vi "WS1050 36 DUT CP CV Sweep SubVI.vi"(0 "TMN DC\\CAP Data Log File Path":path=path "C:/WS1050 36 DUT Data", 1 "Test Program":string="WS1050 36 DUT CP CV Sweep SubVI", 3 "Lot#":string="WS1050", 4 "Wafer#":string="T7-EB", 5 "Board#":string="BRD5", 6 "Temp":string, 7 "error in (no error)":errorcluster, 8 "File Name":string="CYC_WS1050_T7_EB_65C_40V_25DC_EMPTY_BRD5_141017_1", 9 "Comment":string="CYC65C40V", 10 "Ke2400":refnum<visa-resource-name>="GPIB0::3::INSTR", 11 "PS1 Source":refnum<visa-resource-name>="GPIB0::5::INSTR", 12 "Serial Number":string[][](table)=[["DUT", "SN"], ["DUT1", "1"], ["DUT2", "2"], ["DUT3", "3"], ["DUT4", "4"], ["DUT5", "5"], ["DUT6", "6"], ["DUT7", "7"], ["DUT8", "8"], ["DUT9", "9"], ["DUT10", "10"], ["DUT11", "11"], ["DUT12", "12"], ["DUT13", "13"], ["DUT14", "14"], ["DUT15", "15"], ["DUT16", "16"], ["DUT17", "17"], ["DUT18", "18"], ["DUT19", "19"], ["DUT20", "20"], ["DUT21", "21"], ["DUT22", "22"], ["DUT23", "23"], ["DUT24", "24"], ["DUT25", "25"], ["DUT26", "26"], ["DUT27", "27"], ["DUT28", "28"], ["DUT29", "29"], ["DUT30", "30"], ["DUT31", "31"], ["DUT32", "32"], ["DUT33", "33"], ["DUT34", "34"], ["DUT35", "35"], ["DUT36", "36"]], 14 "CP Set to Run":dbl[][](array[numeric]), 16 "HD/Cycles Completed":string="Test Data", 18 "Ke2000":refnum<visa-resource-name>="GPIB0::9::INSTR") -> (13 "40V_1":string[][](table), 15 "40V_2":string[][](table), 17 "40V_3":string[][](table), 20 "Plot_1":dbl[][](graph) caption="(Y) Multi Plot 2", 21 "Plot_2":dbl[][](graph) caption="(Y) Multi Plot 2", 22 "Ke2400 Out":refnum<visa-resource-name>="GPIB0::3::INSTR", 23 "Plot_3":dbl[][](graph) caption="(Y) Multi Plot 2", 24 "CP Voltage":string, 25 "PS1 Out":refnum<visa-resource-name>, 26 "Ke2000 Out":refnum<visa-resource-name>="GPIB0::9::INSTR", 27 "error out":errorcluster)   [LabVIEW 2012]
uses:
  WS_VCAP Driver 029/Source/WSVCAP Shell/Type Defs/WSVCAP SHL I2C DUT Mask Mode Enum.ctl
panel:
  in  "Reg1_Bit Cntrl":string[](array[string])=["01", "02", "04", "08", "10", "20", "40", "80", "03", "06", "0C", "D8", "33", "66", "CC", "07", "0E", "1C", "38", "70", "E0", "0F", "1E", "3C", "78", "F0", "1F", "3E", "7C", "F8", "3F", "7E", "FC", "7F", "FE", "FD", "FB", "F7", "EF", "DF", "BF", "7F", "FC", "F9", "F3", "E7", "CF", "9F", "3F", "F8", "F1", "E3", "C7", "8F", "1F", "F0", "E1", "C3", "87", "0F", "E0", "C1", "83", "07", "C0", "81", "03", "AA", "55", "00"]
  out "date string":string="5/19/2014"
  in  "VPI_Cmd":string[](array[string])=["00", "3B", "00"]
  in  "VPI Name":string[](array[string])=["All_Drivers OFF", "All Drivers ON", "All Drivers OFF2"]
  in  "Tab Control":T1(tab)
  in  "Set VDD":dbl=3.7 format="%.3g"
  in  "Clock Rate (Hz)":dbl=1000000.0 caption="Meas Speed" format="%.1p Hz"
  out "AR  Measurent(Hz)":dbl
  in  "RFFE Slave Address":u8=7 caption="Slave Address" format="0x%02x"
  in  "CP VPI":i32(ring) items=["CP HDC 35V", "CP HDC 40.25V", "CP HDC 27.5V", "CP HDC 30.5V", "CP HDC 44V"]
  in  "Control Panel":T2={"CP C-V \nSweep"=TRUE, "HD/CYC"=FALSE, "E-CAL"=FALSE, "DVA"=FALSE, "VPI"=FALSE, "VSA"=FALSE, "HS"=FALSE}
  out "CP C-V Sweep":bool
  out "HD/CYC":bool
  out "E-CAL":bool
  out "DVA":bool
  out "VPI":bool
  out "VSA":bool
  out "HS":bool
  in  "Freq(Hz)":string="12K"
  in  "Test Sequences":i32(ring) items=["C1_C2_C3", "C2_C1_C3", "C3_C2_C1"]
  in  "WS1050/51":bool=TRUE
  in  "CP with DVA ON":i32(ring) items=["CP HDC 35V", "CP HDC 40.25V", "CP HDC 27.5V", "CP HDC 30.5V", "CP HDC 44V"]
  in  "% Duty Cycle":string="NA"
  in  "Cmin/Act":bool=TRUE
  in  "Current Input":string="71.772763E+0"
  out "NOM IDD OFF(uA)":string
  out "No of HD/Cycle\nCompleted":i32
  out "Loop \ncompleted":i32=1
  out "Previous Time":string="12:20:26 PM"
  out "STATUS":string="Idle...."
  out "Total Delta C2(pF)":string[](array[string])
  out "Total Delta C1(pF)":string[](array[string])
  out "Total Delta C3(pF)":string[](array[string])
  out "RB Reg for HD/Cycle":string[](array[string])
  out "VPI C2":string[][](table)
  out "VPI C3":string[][](table)
  out "NOM IDD ON (uA)":string
  out "IDD_HD/CYC (uA)":string="164.601255E+0"
  out "IDD Stdby(uA)":string="2.606990E+0"
  out "VPI C1":string[][](table)
  out "Loops Run":i64
  out "VSA_V1":string[][](table)
  out "VSA_V2":string[][](table)
  out "VSA_V3":string[][](table)
  in  "VSA Voltage(V)":dbl[](array[numeric])=[-10.0, 0.0, 10.0]
  in  "X Repeat":i32=100
  out "% Delta C_T0":string[][](array[string])
  out "% Delta C":string[][](array[string])
  out "EFuse RB T0":string[](array[string])
  out "Current EFuse Read back":string[](array[string])
  out "EFuse Readback Status":bool[](array[boolean])
  in  "DeltaC Target Setting(pF)":dbl=7.375
  in  "Debug":bool
  in  "No of Rows\nFrom Spread Sheet":i32
  in  "Plot Delta Cmin":bool=TRUE
  in  "Plot":T3(ring)
  in  "Bank 2":i32(ring)=4 items=["C1", "C2", "C3", "D_C1", "D_C2", "D_C3"]
  in  "Bank":i32(ring)=3 items=["C1", "C2", "C3", "D_C1", "D_C2", "D_C3"]
  in  "Bank 3":i32(ring)=5 items=["C1", "C2", "C3", "D_C1", "D_C2", "D_C3"]
  # "Company:  WiSpry Inc\n20 Fairbanks Ste 198 Irvine CA 92618\n\nAuthor:  Andy V Tran\nCreated:  08/21/2015\nLabVIEW 2012 Pro\nTest Program:  WS1050 36 DUT CP CV Sweep SubVI\nFPGA: WS_VCAP Driver 029"
  # "Note for HD Duty Cycle:\n1.  Set time to start HD_DC (Min), default is 259200 (6 months) \n2.  Set Time for Duty Cycle ON/OFF, default setting is 2 minutes\n3.  No of Loops to RP = 3600s/(Time ALL ON(s) + Time ALL + OFF(s))\n4.  Set X Repeat = no of runs, default is 100 runs\n5.  Set TTF Completed to stop the test.\n\nVer 1.1 updated based on Ver1.0:\n1.  Updated the control panel ( CP C-V Sweep was set \"Yes\" by default)\n2.  CP Voltage sweep should be set up from look up table."
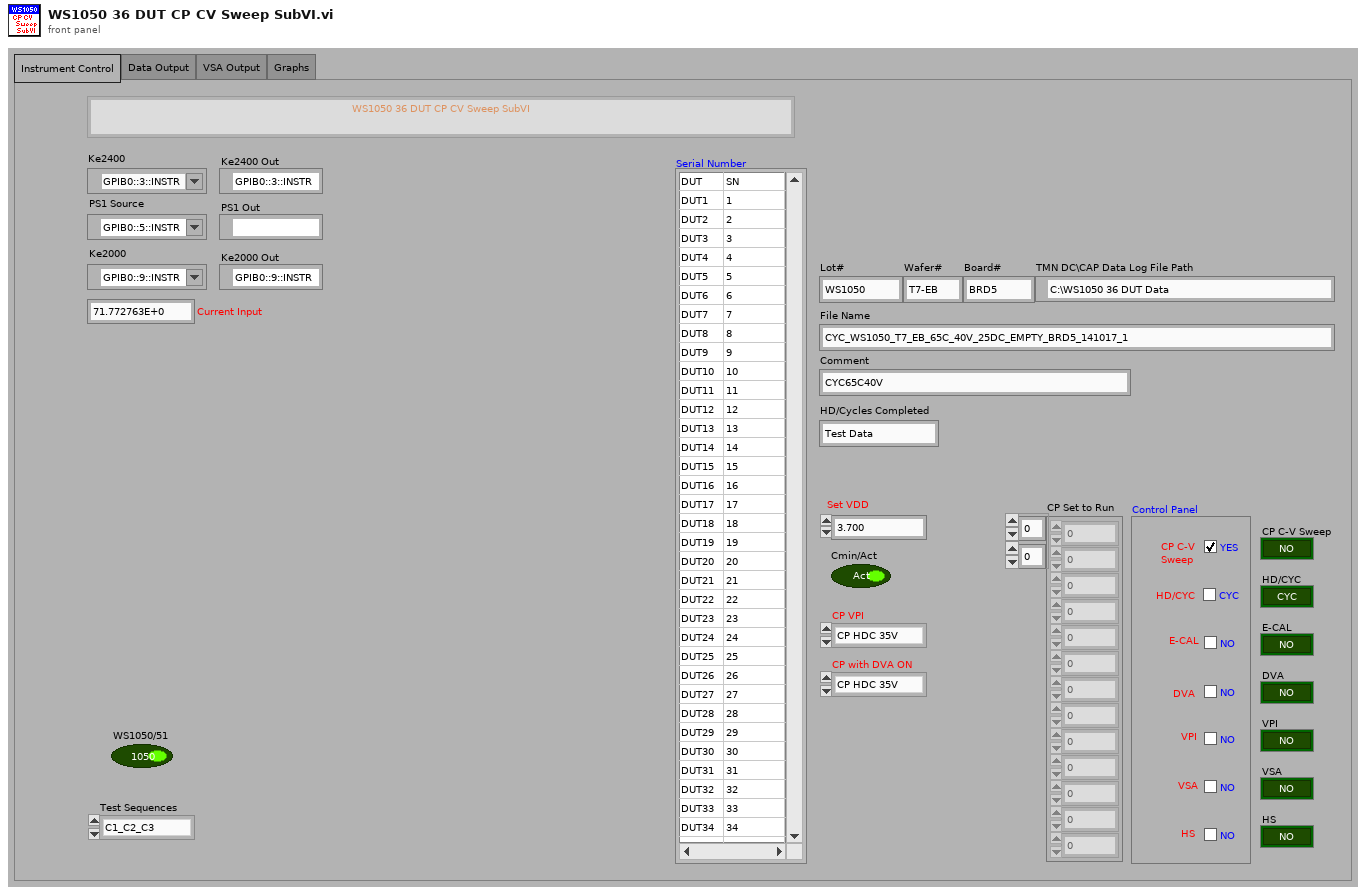
[diagram p1: front panel]
types:
  T1 = enum32{"Instrument Control", "Data Output", "VSA Output", "Graphs"}
  T2 = cluster{"CP C-V \nSweep":bool, "HD/CYC":bool, "E-CAL":bool, "DVA":bool, "VPI":bool, "VSA":bool, "HS":bool}
  T3 = enum16{"ALL DUTs", "DUT 01", "DUT 02", "DUT 03", "DUT 04", "DUT 05", "DUT 06", "DUT 07", "DUT 08", "DUT 09", "DUT 10", "DUT 11", "DUT 12", "DUT 13", "DUT 14", "DUT 15", "DUT 16", "DUT 17", "DUT 18", "DUT 19", "DUT 20", "DUT 21", "DUT 22", "DUT 23", "DUT 24", "DUT 25", "DUT 26", "DUT 27", "DUT 28", "DUT 29", "DUT 30", "DUT 31", "DUT 32", "DUT 33", "DUT 34", "DUT 35", "DUT 36"}
  T4 = typedef "WSVCAP SHL I2C DUT Mask Mode Enum.ctl" = enum16{"Custom", "C1", "C2", "C3", "All"}
  T5 = enum16{"Idle...", "Voltage 1", "Voltage 2", "Voltage 3"}[]
  T6 = cluster{"Test Program ":string, "Comment":string, "Data Out":string, "Data Out":string, "CP Voltage":string, string, "% Duty Cycle":string, "CP Voltage":string, "string":string, "Freq(Hz)":string, "Board#":string}
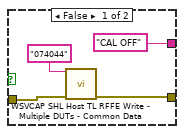
[diagram p3: hidden frame]
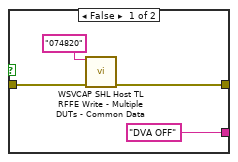
[diagram p4: hidden frame]
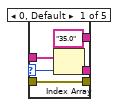
[diagram p5: hidden frame]
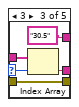
[diagram p6: hidden frame]
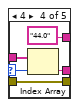
[diagram p7: hidden frame]
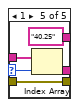
[diagram p8: hidden frame]
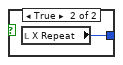
[diagram p9: hidden frame]
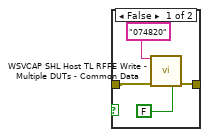
[diagram p10: hidden frame]
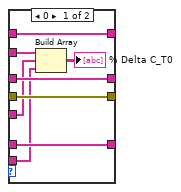
[diagram p11: hidden frame]
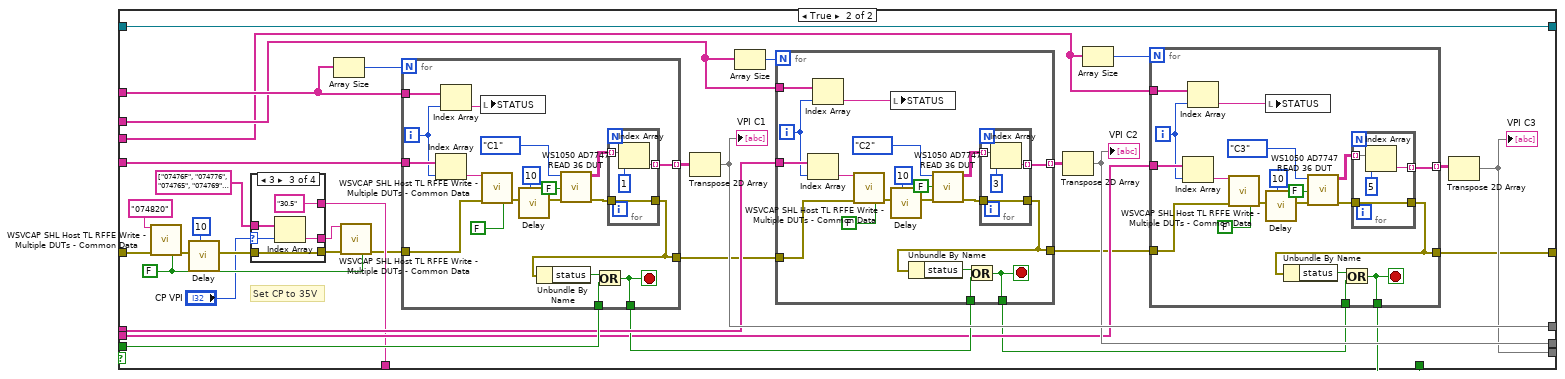
[diagram p12: hidden frame]
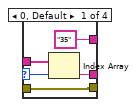
[diagram p13: hidden frame]
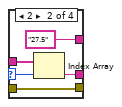
[diagram p14: hidden frame]
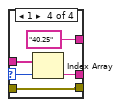
[diagram p15: hidden frame]
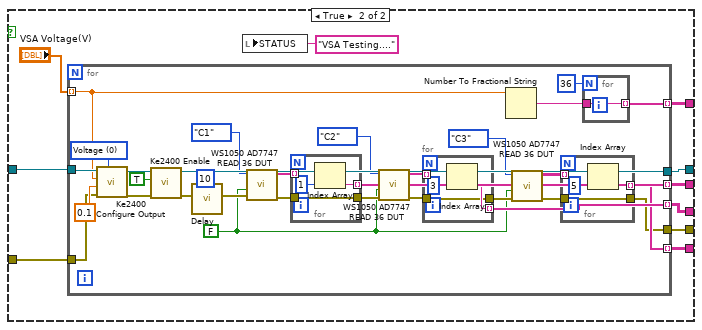
[diagram p17: hidden frame]
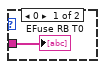
[diagram p18: hidden frame]
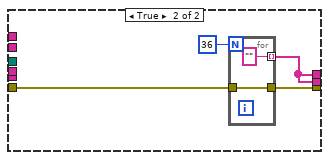
[diagram p19: hidden frame]
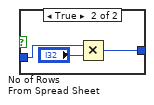
[diagram p20: hidden frame]
diagram:
  n1 = call "WSVCAP SHL Host TL RFFE Configure.vi"("RFFE Slave Address"="RFFE Slave Address", "Clock Rate (Hz)"="Clock Rate (Hz)", "error in"="error in (no error)") -> ("error out"=w4:errorcluster)  [unwired: 11 in, 1 out]
  n2 = call "Control Panel.vi"("error in (no error)"=w4, "Control Panel"="Control Panel") -> ("error out"=w12:errorcluster, "VPI"=w8:bool, "DVA"=w9:bool, "E-CAL"=w10:bool, "VSA"=w7:bool, "HD/CYC"=w11:bool, "HS"=w6:bool, "Verify Socket"=w1:bool)  [unwired: 2 in]
  "CP C-V Sweep" <- w1
  "E-CAL" <- w10
  "VPI" <- w8
  "VSA" <- w7
  "HS" <- w6
  "HD/CYC" <- w11
  "DVA" <- w9
  n3 = case shown="True" w1 {
    tunnel: w12 -> [w26 w77]
    tunnel: [w26 w28] -> w15
    tunnel: "CP Set to Run" -> [_ w78]
    tunnel: "PS1 Source" -> [w24 w76]
    tunnel: "Ke2000" -> [w25 w70]
    tunnel: [w25 w74] -> w22
    tunnel: [w24 w29] -> w21
    tunnel: "Ke2400" -> [w23 w67]
    tunnel: [w23 w64] -> w16
    tunnel: "RFFE Slave Address" -> [_ w61]
    tunnel: w11 -> [_ w40]
    tunnel: w10 -> [_ w39]
    tunnel: w9 -> [_ w38]
    tunnel: w8 -> [_ w37]
    tunnel: w7 -> [_ w36]
    tunnel: w6 -> [_ w35]
    tunnel: "Clock Rate (Hz)" -> [_ w27]
    frame False {
    }
    frame True {
      w45 = u32 100 ("milliseconds to wait")
      w75 = T5 [enum."Voltage 2", enum."Voltage 3", enum."Voltage 1"] items=["Idle...", "Voltage 1", "Voltage 2", "Voltage 3"]
      # "VSA"
      # "HS"
      # "HD/CYC"
      # "DVA"
      # "E-CAL"
      # "VPI"
      n4 = for {
        tunnel: w77 -> [w1121]
        tunnel: w76 -> [w1120]
        tunnel: w75 -> [w1118] mode=indexing
        tunnel: [w1113] -> w72
        tunnel: [w1117] -> w63
        n5 = local read "Set VDD"() -> (w1116:dbl)
        n6 = call "E3631A_Voltage Controller updated.vi"("VISA resource name"=w1120, "I_VDD(A)"=0.5, "Channel Controller"=w1118, "Voltage 1"=w1116, "Voltage 2"=3.3, "error in (no error)"=w1121, "I_3.3V (A)"=0.5) -> ("VISA resource name out"=w1117:refnum<visa-resource-name>, "error out"=w1114:errorcluster)  [unwired: 7 in]
        n7 = call "Delay.vi"("milliseconds to wait"=u32 100, "error in (no error)"=w1114) -> ("error out"=w1113:errorcluster)  [unwired: 9 in]
      }
      n8 = call "WSVCAP SHL Host TL RFFE Write - Multiple DUTs - Common Data.vi"("Data Out"="074000", "error in"=w72, "Log (T)"=FALSE) -> ("error out"=w73:errorcluster)  [unwired: 12 in]
      n9 = call "Delay.vi"("milliseconds to wait"=w45, "error in (no error)"=w73) -> ("error out"=w71:errorcluster)  [unwired: 9 in]
      n10 = call "Ke2000 Single Reading.vi"("error in (no error)"=w71, "VISA resource name"=w70) -> ("error out"=w51:errorcluster, "VISA resource name out"=w69:refnum<visa-resource-name>, "uA"=w53:string)  [unwired: 5 in, 2 out]
      n11 = call "Substration.vi"("error in (no error)"=w51, "Input2"="Current Input", "Input1"=w53) -> ("error out"=w32:errorcluster, "In1 - In2"=w52:string)  [unwired: 7 in]
      "IDD Stdby(uA)" <- w52
      n12 = case shown="False" w40 {
        tunnel: [1 ("X Repeat") w139] -> w62
        frame False {
        }
        frame True {
          n13 = local read "X Repeat"() -> (w139:i32)
        }
      }
      n14 = call "WSVCAP SHL Host TL RFFE Write - Multiple DUTs - Common Data.vi"("Data Out"="074040", "error in"=w32, "Log (T)"=FALSE) -> ("error out"=w31:errorcluster)  [unwired: 12 in]
      n15 = call "Delay.vi"("milliseconds to wait"=w45, "error in (no error)"=w31) -> ("error out"=w59:errorcluster)  [unwired: 9 in]
      n16 = case shown="True" w38 {
        tunnel: w59 -> [w101 w110]
        tunnel: [w100 w108] -> w57
        tunnel: ["DVA OFF" ("Data Out") "DVA ON" ("Data Out")] -> w58
        frame False {
          n17 = call "WSVCAP SHL Host TL RFFE Write - Multiple DUTs - Common Data.vi"("Data Out"="074820", "error in"=w101) -> ("error out"=w100:errorcluster)  [unwired: 13 in]
        }
        frame True {
          n18 = call "WSVCAP SHL Host TL RFFE Write - Multiple DUTs - Common Data.vi"("Data Out"="074800", "error in"=w110, "Log (T)"=FALSE) -> ("error out"=w106:errorcluster)  [unwired: 12 in]
          n19 = case shown="2" "CP with DVA ON" {
            selector: "CP with DVA ON" -> [w116 w121 w126 w131 w135]
            tunnel: string[] ["07442F", "074436", "074428", "074429", "07443B"] -> [w117 w122 w127 w132 w137]
            tunnel: [w115 w120 w125 w130 w136] -> w102
            tunnel: ["35.0" ("Data Out") "29.75" ("Data Out") "30.5" ("Data Out") "44.0" ("Data Out") "40.25" ("Data Out")] -> _
            tunnel: w106 -> [w113 w118 w123 w128 w133]
            tunnel: [w113 w118 w123 w128 w133] -> w105
            frame 0, Default {
              n20 = Index Array(array=w117, index=w116) -> (element=w115:string)
            }
            frame 2 {
              n21 = Index Array(array=w122, index=w121) -> (element=w120:string)
            }
            frame 3 {
              n22 = Index Array(array=w127, index=w126) -> (element=w125:string)
            }
            frame 4 {
              n23 = Index Array(array=w132, index=w131) -> (element=w130:string)
            }
            frame 1 {
              n24 = Index Array(array=w137, index=w135) -> (element=w136:string)
            }
          }
          n25 = call "WSVCAP SHL Host TL RFFE Write - Multiple DUTs - Common Data.vi"("Data Out"=w102, "error in"=w105, "Log (T)"=FALSE) -> ("error out"=w108:errorcluster)  [unwired: 12 in]
        }
      }
      n26 = for {
        N: 36 -> [_]
        tunnel: "Serial Number" -> [w83]
        tunnel: [w81] -> w42 mode=indexing
        i -> [w80]
        n27 = Increment(x=w80) -> (x+1=w79:i32)
        n28 = Index Array(array=w83, index (row)=w79, index (col)=1 ("disabled index (col)")) -> (element=w81:string)
      }
      n29 = Not(x=w35) -> (.not. x?=w41:bool)
      n30 = Number To Fractional String(number="Set VDD", precision (6)=i16 2) -> (F-format string=w55:string)  [unwired: 2 in]
      n31 = call "Delay.vi"("milliseconds to wait"=w45, "error in (no error)"=w57) -> ("error out"=w48:errorcluster)  [unwired: 9 in]
      n32 = case shown="True" w39 {
        tunnel: w48 -> [w87 w89]
        tunnel: [w84 w88] -> w47
        tunnel: ["CAL OFF" ("Data Out") "CAL ON" ("Data Out")] -> w49
        frame False {
          n33 = call "WSVCAP SHL Host TL RFFE Write - Multiple DUTs - Common Data.vi"("Data Out"="074044", "error in"=w87) -> ("error out"=w84:errorcluster)  [unwired: 13 in]
        }
        frame True {
          n34 = for {
            tunnel: string[] ["074900", "074920", "074900"] -> [w97] mode=indexing
            tunnel: w89 -> [w94]
            tunnel: [w93] -> w88
            n35 = call "WSVCAP SHL Host TL RFFE Write - Multiple DUTs - Common Data.vi"("Data Out"=w97, "error in"=w94, "Log (T)"=FALSE) -> ("error out"=w96:errorcluster)  [unwired: 12 in]
            n36 = call "Delay.vi"("milliseconds to wait"=u32 10, "error in (no error)"=w96) -> ("error out"=w93:errorcluster)  [unwired: 9 in]
          }
        }
      }
      n37 = for {
        N: w62 -> [_]
        tunnel: w78 -> [w168]
        tunnel: [w164] -> w74
        tunnel: w52 -> [w163]
        tunnel: w69 -> [w162]
        tunnel: "TMN DC\\CAP Data Log File Path" -> [w161]
        tunnel: w67 -> [w159]
        tunnel: [w158] -> w65
        tunnel: w63 -> [w143]
        tunnel: w61 -> [w154]
        tunnel: w58 -> [w153]
        tunnel: w55 -> [w152]
        tunnel: [w151] -> w50
        tunnel: w49 -> [w150]
        tunnel: w47 -> [w149]
        tunnel: w38 -> [w148]
        tunnel: w37 -> [w147]
        tunnel: w41 -> [w146]
        tunnel: w36 -> [w145]
        tunnel: w42 -> [w144]
        tunnel: [w143] -> w29
        tunnel: "Current Input" -> [w142]
        tunnel: w27 -> [w140]
        stop <- w141 stop-if-true
        (unwired) u64 0
        n38 = while {
          tunnel: w168 -> [w186]
          tunnel: w161 -> [w387]
          tunnel: "Lot#" -> [w386]
          tunnel: "Wafer#" -> [w385]
          tunnel: w144 -> [w384]
          tunnel: "Test Program" -> [w383]
          tunnel: w144 -> [w382]
          tunnel: "Comment" -> [w381]
          tunnel: "Lot#" -> [w380]
          tunnel: "Wafer#" -> [w379]
          tunnel: w162 -> [w376]
          tunnel: [w378] -> w164
          tunnel: w163 -> [w375]
          tunnel: w159 -> [w373]
          tunnel: [w372] -> w158
          tunnel: [w297] -> w155
          tunnel: w154 -> [w296]
          tunnel: w153 -> [w246]
          tunnel: w152 -> [w244]
          tunnel: [w226] -> w151
          tunnel: w150 -> [w231]
          tunnel: w149 -> [w187]
          tunnel: w148 -> [w230]
          tunnel: w147 -> [w223]
          tunnel: w146 -> [w218]
          tunnel: w145 -> [w212]
          tunnel: w142 -> [w172]
          tunnel: w140 -> [w171]
          i -> [w191]
          stop <- w326 stop-if-true
          n39 = Array Size(array=w186) -> (size(s)=w185:i32[])
          n40 = Index Array(array=w186, index (row)=w191, index (col)=0 ("disabled index (col)")) -> (element=w183:dbl)
          n41 = Index Array(array=w185, index=0) -> (element=w174:i32)
          n42 = call "CP_Cmd_Setting.vi"("error in (no error)"=w187, "Input"=w183) -> ("error out"=w190:errorcluster, "CP Voltage"=w188:string, "Send Cmd"=w189:string)  [unwired: 6 in, 1 out]
          "CP Voltage" <- w188
          n43 = To Quad Integer(1:w174) -> (0:w173:i64)
          n44 = flat-sequence {
            tunnel: [w440] -> w371
            tunnel: w376 -> [w429]
            tunnel: w375 -> [w441]
            tunnel: [w441] -> w370
            tunnel: [w406] -> w369
            tunnel: [w403] -> w368
            tunnel: w190 -> [w438]
            tunnel: w191 -> [w388]
            tunnel: [w388] -> w325
            tunnel: ["Temp"] -> w320
            tunnel: [w411] -> w315
            tunnel: [w410] -> w314
            tunnel: [w409] -> w313
            tunnel: [w415] -> w303
            tunnel: [w412] -> w302
            tunnel: w296 -> [w437]
            tunnel: [w437] -> w295
            tunnel: [w414] -> w283
            tunnel: [w413] -> w259
            tunnel: [w389] -> w247
            tunnel: w189 -> [w435]
            tunnel: ["% Duty Cycle"] -> w243
            tunnel: [w396] -> w235
            tunnel: w223 -> [w424]
            tunnel: [w424] -> w222
            tunnel: w218 -> [w423]
            tunnel: [w423] -> w217
            tunnel: w212 -> [w422]
            tunnel: [w422] -> w211
            tunnel: [w418] -> w206
            tunnel: ["WS1050/51"] -> w200
            tunnel: ["Cmin/Act"] -> w196
            tunnel: w173 -> [w394]
            tunnel: w183 -> [w395]
            tunnel: [w394] -> w182
            tunnel: w172 -> [w393]
            tunnel: w171 -> [w389]
            tunnel: [w493] -> w294
            tunnel: w371 -> [w496]
            tunnel: w370 -> [w499]
            tunnel: w369 -> [w495]
            tunnel: w368 -> [w494]
            tunnel: [w484] -> w293
            tunnel: [w499] -> w292
            tunnel: [w495] -> w291
            tunnel: [w494] -> w290
            tunnel: w325 -> [w498]
            tunnel: [w498] -> w289
            tunnel: w320 -> [w497]
            tunnel: [w497] -> w288
            tunnel: [w496] -> w287
            tunnel: w315 -> [w492]
            tunnel: w314 -> [w477]
            tunnel: w313 -> [w478]
            tunnel: [w489] -> w286
            tunnel: w303 -> [w491]
            tunnel: w302 -> [w489]
            tunnel: [w485] -> w285
            tunnel: w295 -> [w490]
            tunnel: [w475] -> w284
            tunnel: w283 -> [w475]
            tunnel: [w477] -> w282
            tunnel: w259 -> [w476]
            tunnel: [w476] -> w258
            tunnel: [w478] -> w256
            tunnel: w247 -> [w488]
            tunnel: [w487] -> w236
            tunnel: w235 -> [w487]
            tunnel: w222 -> [w483]
            tunnel: [w483] -> w221
            tunnel: w217 -> [w482]
            tunnel: [w482] -> w216
            tunnel: w211 -> [w481]
            tunnel: [w481] -> w210
            tunnel: w206 -> [w480]
            tunnel: [w479] -> w205
            tunnel: w200 -> [w473]
            tunnel: [w473] -> w199
            tunnel: w196 -> [w472]
            tunnel: [w472] -> w195
            tunnel: w182 -> [w471]
            tunnel: [w471] -> w181
            tunnel: w294 -> [w538]
            tunnel: [w537] -> w281
            tunnel: w293 -> [w529]
            tunnel: [w529] -> w278
            tunnel: w292 -> [w548]
            tunnel: [w548] -> w276
            tunnel: w291 -> [w547]
            tunnel: [w547] -> w274
            tunnel: w290 -> [w546]
            tunnel: [w546] -> w272
            tunnel: w289 -> [w545]
            tunnel: [w545] -> w270
            tunnel: w288 -> [w544]
            tunnel: [w544] -> w268
            tunnel: w287 -> [w543]
            tunnel: [w543] -> w266
            tunnel: w286 -> [w542]
            tunnel: [w542] -> w264
            tunnel: [w534] -> w262
            tunnel: w285 -> [w533]
            tunnel: w284 -> [w540]
            tunnel: w282 -> [w539]
            tunnel: w258 -> [w526]
            tunnel: [w526] -> w257
            tunnel: w256 -> [w528]
            tunnel: [w528] -> w255
            tunnel: [w535] -> w254
            tunnel: [w536] -> w237
            tunnel: w236 -> [w536]
            tunnel: w221 -> [w532]
            tunnel: [w532] -> w220
            tunnel: w216 -> [w531]
            tunnel: [w531] -> w215
            tunnel: w210 -> [w530]
            tunnel: [w530] -> w209
            tunnel: w205 -> [w527]
            tunnel: [w527] -> w202
            tunnel: w199 -> [w524]
            tunnel: [w524] -> w198
            tunnel: w195 -> [w523]
            tunnel: [w523] -> w194
            tunnel: w181 -> [w522]
            tunnel: [w522] -> w180
            tunnel: w281 -> [w588]
            tunnel: [w587] -> w280
            tunnel: [w583] -> w279
            tunnel: w278 -> [w577]
            tunnel: [w577] -> w277
            tunnel: w276 -> [w599]
            tunnel: [w599] -> w275
            tunnel: w274 -> [w598]
            tunnel: [w598] -> w273
            tunnel: w272 -> [w597]
            tunnel: [w597] -> w271
            tunnel: w270 -> [w596]
            tunnel: [w596] -> w269
            tunnel: w268 -> [w595]
            tunnel: [w595] -> w267
            tunnel: w266 -> [w594]
            tunnel: [w594] -> w265
            tunnel: w264 -> [w593]
            tunnel: [w593] -> w263
            tunnel: w262 -> [w592]
            tunnel: [w592] -> w261
            tunnel: [w575] -> w260
            tunnel: w257 -> [w590]
            tunnel: w255 -> [w589]
            tunnel: w254 -> [w582]
            tunnel: ["DeltaC Target Setting(pF)"] -> w245
            tunnel: [w585] -> w238
            tunnel: w237 -> [w585]
            tunnel: w230 -> [w584]
            tunnel: [w584] -> w229
            tunnel: w220 -> [w581]
            tunnel: [w581] -> w219
            tunnel: w215 -> [w580]
            tunnel: [w580] -> w214
            tunnel: w209 -> [w579]
            tunnel: [w579] -> w208
            tunnel: w202 -> [w578]
            tunnel: [w575] -> w201
            tunnel: w198 -> [w574]
            tunnel: [w574] -> w197
            tunnel: w194 -> [w573]
            tunnel: [w573] -> w193
            tunnel: w180 -> [w572]
            tunnel: [w572] -> w179
            tunnel: [w677] -> w367
            tunnel: [w643] -> w366
            tunnel: w280 -> [w680]
            tunnel: w279 -> [w657]
            tunnel: [w666] -> w365
            tunnel: [w657] -> w364
            tunnel: [w679] -> w363
            tunnel: [w678] -> w362
            tunnel: w277 -> [w666]
            tunnel: w275 -> [w676]
            tunnel: [w676] -> w361
            tunnel: w273 -> [w672]
            tunnel: [w672] -> w360
            tunnel: w271 -> [w671]
            tunnel: [w671] -> w359
            tunnel: w269 -> [w667]
            tunnel: [w667] -> w324
            tunnel: w267 -> [w675]
            tunnel: [w675] -> w319
            tunnel: w265 -> [w674]
            tunnel: [w673] -> w316
            tunnel: w263 -> [w669]
            tunnel: w261 -> [w665]
            tunnel: [w670] -> w312
            tunnel: [w668] -> w311
            tunnel: [w665] -> w306
            tunnel: w260 -> [w664]
            tunnel: [w651] -> w301
            tunnel: [w650] -> w300
            tunnel: [w649] -> w299
            tunnel: w245 -> [w663]
            tunnel: [w648] -> w239
            tunnel: w238 -> [w648]
            tunnel: [w647] -> w234
            tunnel: w229 -> [w646]
            tunnel: w219 -> [w641]
            tunnel: w214 -> [w640]
            tunnel: [w640] -> w213
            tunnel: w208 -> [w639]
            tunnel: [w639] -> w207
            tunnel: w201 -> [w636]
            tunnel: w197 -> [w635]
            tunnel: w193 -> [w624]
            tunnel: w179 -> [w623]
            tunnel: [w623] -> w178
            tunnel: w367 -> [w883]
            tunnel: [w883] -> w358
            tunnel: [w869] -> w357
            tunnel: [w882] -> w356
            tunnel: w366 -> [w881]
            tunnel: w365 -> [w880]
            tunnel: w364 -> [w879]
            tunnel: [w880] -> w355
            tunnel: [w879] -> w354
            tunnel: w363 -> [w878]
            tunnel: [w878] -> w353
            tunnel: w362 -> [w877]
            tunnel: [w877] -> w352
            tunnel: w361 -> [w876]
            tunnel: [w876] -> w351
            tunnel: w360 -> [w875]
            tunnel: [w875] -> w350
            tunnel: w359 -> [w874]
            tunnel: [w874] -> w349
            tunnel: w373 -> [w873]
            tunnel: [w871] -> w348
            tunnel: [w851] -> w347
            tunnel: [w852] -> w346
            tunnel: [w850] -> w345
            tunnel: w324 -> [w867]
            tunnel: [w867] -> w323
            tunnel: w319 -> [w866]
            tunnel: [w866] -> w318
            tunnel: w316 -> [w882]
            tunnel: w312 -> [w864]
            tunnel: w311 -> [w865]
            tunnel: [w865] -> w310
            tunnel: [w864] -> w308
            tunnel: w306 -> [w863]
            tunnel: [w863] -> w305
            tunnel: w301 -> [w849]
            tunnel: w300 -> [w848]
            tunnel: w299 -> [w847]
            tunnel: [w844] -> w298
            tunnel: [w849] -> w253
            tunnel: [w848] -> w251
            tunnel: [w847] -> w249
            tunnel: [w846] -> w240
            tunnel: w239 -> [w846]
            tunnel: w234 -> [w845]
            tunnel: [w845] -> w233
            tunnel: w213 -> [w844]
            tunnel: w207 -> [w843]
            tunnel: w178 -> [w842]
            tunnel: [w842] -> w177
            tunnel: w358 -> [w977]
            tunnel: [w977] -> w344
            tunnel: w357 -> [w998]
            tunnel: [w997] -> w343
            tunnel: w387 -> [w999]
            tunnel: w386 -> [w996]
            tunnel: w385 -> [w995]
            tunnel: w384 -> [w994]
            tunnel: [w993] -> w342
            tunnel: w356 -> [w987]
            tunnel: [w987] -> w341
            tunnel: w355 -> [w992]
            tunnel: w354 -> [w991]
            tunnel: [w992] -> w340
            tunnel: [w991] -> w339
            tunnel: [w985] -> w338
            tunnel: w353 -> [w990]
            tunnel: [w990] -> w337
            tunnel: w352 -> [w989]
            tunnel: [w989] -> w336
            tunnel: [w988] -> w335
            tunnel: w351 -> [w986]
            tunnel: w350 -> [w984]
            tunnel: w349 -> [w983]
            tunnel: "File Name" -> [w982]
            tunnel: w348 -> [w981]
            tunnel: [w981] -> w334
            tunnel: w347 -> [w980]
            tunnel: [w980] -> w333
            tunnel: [w979] -> w332
            tunnel: w346 -> [w979]
            tunnel: w345 -> [w978]
            tunnel: [w978] -> w331
            tunnel: w323 -> [w961]
            tunnel: [w961] -> w321
            tunnel: w318 -> [w975]
            tunnel: [w975] -> w317
            tunnel: w310 -> [w974]
            tunnel: [w974] -> w309
            tunnel: w308 -> [w973]
            tunnel: [w973] -> w307
            tunnel: w305 -> [w972]
            tunnel: [w972] -> w304
            tunnel: w298 -> [w971]
            tunnel: w253 -> [w970]
            tunnel: [w970] -> w252
            tunnel: w251 -> [w969]
            tunnel: [w969] -> w250
            tunnel: w249 -> [w968]
            tunnel: [w968] -> w248
            tunnel: w243 -> [w967]
            tunnel: [w967] -> w242
            tunnel: [w966] -> w241
            tunnel: w240 -> [w966]
            tunnel: w233 -> [w965]
            tunnel: [w965] -> w232
            tunnel: ["Freq(Hz)"] -> w204
            tunnel: ["Board#"] -> w203
            tunnel: w177 -> [w962]
            tunnel: [w962] -> w176
            tunnel: ["Debug"] -> w170
            tunnel: w344 -> [w1072]
            tunnel: w343 -> [w1071]
            tunnel: w387 -> [w1037]
            tunnel: w383 -> [w1066]
            tunnel: w382 -> [w1069]
            tunnel: w381 -> [w1065]
            tunnel: w380 -> [w1068]
            tunnel: w379 -> [w1064]
            tunnel: w342 -> [w1067]
            tunnel: [w1072] -> w328
            tunnel: [w1070] -> w329
            tunnel: w341 -> [w1062]
            tunnel: [w1062] -> w330
            tunnel: w340 -> [w1061]
            tunnel: w339 -> [w1049]
            tunnel: w338 -> [w1060]
            tunnel: w337 -> [w1059]
            tunnel: w336 -> [w1051]
            tunnel: w335 -> [w1058]
            tunnel: "File Name" -> [w1031]
            tunnel: w334 -> [w1057]
            tunnel: [w1057] -> w327
            tunnel: w333 -> [w1056]
            tunnel: w332 -> [w1055]
            tunnel: w331 -> [w1054]
            tunnel: [w1033] -> w322
            tunnel: w321 -> [w1033]
            tunnel: w317 -> [w1053]
            tunnel: w309 -> [w1052]
            tunnel: w307 -> [w1050]
            tunnel: w304 -> [w1048]
            tunnel: w252 -> [w1047]
            tunnel: w250 -> [w1046]
            tunnel: w248 -> [w1045]
            tunnel: w246 -> [w1044]
            tunnel: w231 -> [w1043]
            tunnel: w188 -> [w1042]
            tunnel: w244 -> [w1041]
            tunnel: w242 -> [w1040]
            tunnel: w241 -> [w1039]
            tunnel: w232 -> [w1038]
            tunnel: [w1035] -> w228
            tunnel: [w1028] -> w224
            tunnel: w204 -> [w1027]
            tunnel: w203 -> [w1025]
            tunnel: w176 -> [w1024]
            tunnel: [w1024] -> w175
            tunnel: w170 -> [w1022]
            tunnel: [w1091] -> w377
            tunnel: [w1092] -> w378
            tunnel: [w1093] -> w297
            tunnel: w330 -> [w1092]
            tunnel: w329 -> [w1085]
            tunnel: w328 -> [w1093]
            tunnel: w327 -> [w1086]
            tunnel: [w1086] -> w372
            tunnel: w322 -> [w1078]
            tunnel: [w1084] -> w225
            tunnel: w228 -> [w1083]
            tunnel: w224 -> [w1081]
            tunnel: w175 -> [w1080]
            tunnel: [w1077] -> w169
            frame #0 {
              w419 = FALSE ("Log (T)")
              n45 = call "WSVCAP SHL Host TL RFFE Write - Multiple DUTs - Common Data.vi"("Data Out"=w435, "error in"=w438, "Log (T)"=FALSE) -> ("error out"=w425:errorcluster)  [unwired: 12 in]
              n46 = for {
                tunnel: string[] ["0760", "0767", "0768"] -> [w463] mode=indexing
                tunnel: [w459] -> w427 mode=indexing
                tunnel: w425 -> [w457]
                tunnel: [w456] -> w426
                i -> [w462]
                n47 = call "Delay.vi"("milliseconds to wait"=u32 10, "error in (no error)"=w457) -> ("error out"=w464:errorcluster)  [unwired: 9 in]
                n48 = call "WSVCAP SHL Host TL RFFE Read - Multiple DUTs - Common Data.vi"("Data Out"=w463, "error in"=w464, "Log (T)"=FALSE) -> ("RFFE Data In"=w461:string[], "error out"=w456:errorcluster)  [unwired: 11 in]
                n49 = Index Array(array=w461, index=w462) -> (element=w458:string)
                n50 = String Subset(string=w458, offset (0)=0) -> (substring=w459:string)  [unwired: 1 in]
              }
              "RB Reg for HD/Cycle" <- w427
              n51 = call "Delay.vi"("milliseconds to wait"=u32 100, "error in (no error)"=w426) -> ("error out"=w431:errorcluster)  [unwired: 9 in]
              n52 = call "Ke2000 Single Reading.vi"("error in (no error)"=w431, "VISA resource name"=w429) -> ("error out"=w433:errorcluster, "VISA resource name out"=w408:refnum<visa-resource-name>, "uA"=w434:string)  [unwired: 5 in, 2 out]
              n53 = call "Substration.vi"("error in (no error)"=w433, "Input2"=w393, "Input1"=w434) -> ("error out"=w390:errorcluster, "In1 - In2"=→"IDD_HD/CYC (uA)":string)  [unwired: 7 in]
              n54 = call "CP_Cmd_Setting.vi"("error in (no error)"=w390, "Input"=w395) -> ("error out"=w398:errorcluster, "CP Voltage"=w396:string, "Send Cmd"=w397:string)  [unwired: 6 in, 1 out]
              n55 = call "WSVCAP SHL Host TL RFFE Write - Multiple DUTs - Common Data.vi"("Data Out"=w397, "error in"=w398, "Log (T)"=w419) -> ("error out"=w436:errorcluster)  [unwired: 12 in]
              n56 = flat-sequence {
                tunnel: w421 -> [w466]
                tunnel: [w466] -> w417
                frame #0 {
                  w467 = "0" ("NOM IDD OFF(uA)")
                  w468 = string[] []
                  w469 = string[][] []
                  n57 = local write "Total Delta C1(pF)"(w468) -> ()
                  n58 = local write "Total Delta C2(pF)"(w468) -> ()
                  n59 = local write "Total Delta C3(pF)"(w468) -> ()
                  n60 = local write "Current EFuse Read back"(w468) -> ()
                  n61 = local write "NOM IDD ON (uA)"(w467) -> ()
                  n62 = local write "NOM IDD OFF(uA)"(w467) -> ()
                  n63 = local write "VSA_V3"(w469) -> ()
                  n64 = local write "VSA_V1"(w469) -> ()
                  n65 = local write "VSA_V2"(w469) -> ()
                  n66 = local write "VPI C1"(w469) -> ()
                  n67 = local write "VPI C2"(w469) -> ()
                  n68 = local write "VPI C3"(w469) -> ()
                  n69 = local write "% Delta C"(w469) -> ()
                  n70 = local write "40V_3"(w469) -> ()
                  n71 = local write "40V_2"(w469) -> ()
                  n72 = local write "40V_1"(w469) -> ()
                }
              }
              n73 = call "Delay.vi"("milliseconds to wait"=u32 50, "error in (no error)"=w436) -> ("error out"=w401:errorcluster)  [unwired: 9 in]
              n74 = for {
                tunnel: [w454] -> w440
                tunnel: [w453] -> w421
                tunnel: w419 -> [w452]
                tunnel: w408 -> [w451]
                tunnel: w401 -> [w447]
                tunnel: string[] ["0702013B3B3B", "070201000000"] -> [w444] mode=indexing
                tunnel: [w443] -> w404 mode=indexing
                tunnel: w393 -> [w442]
                n75 = call "WSVCAP SHL Host TL RFFE Write - Multiple DUTs - Common Data.vi"("Data Out"=w444, "error in"=w447, "Log (T)"=w452) -> ("error out"=w448:errorcluster)  [unwired: 12 in]
                n76 = call "Delay.vi"("milliseconds to wait"=u32 100, "error in (no error)"=w448) -> ("error out"=w449:errorcluster)  [unwired: 9 in]
                n77 = call "Ke2000 Single Reading.vi"("error in (no error)"=w449, "VISA resource name"=w451) -> ("error out"=w446:errorcluster, "VISA resource name out"=w454:refnum<visa-resource-name>, "uA"=w445:string)  [unwired: 5 in, 2 out]
                n78 = call "Substration.vi"("error in (no error)"=w446, "Input2"=w442, "Input1"=w445) -> ("error out"=w453:errorcluster, "In1 - In2"=w443:string)  [unwired: 7 in]
              }
              n79 = Index Array(array=w404, index=0) -> (element=w406:string)
              n80 = Index Array(array=w404, index=1) -> (element=w403:string)
              n81 = call "Multi Dut Cmd_Header Setting.vi"("WS1050/51"="WS1050/51", "Cmin/Act"="Cmin/Act", "Test Seq"="Test Sequences", "error in (no error)"=w417) -> ("Name 1"=w415:string[], "Name 2"=w414:string[], "Name Header"=w412:string[], "Name 3"=w413:string[], "Cmd 3"=w409:string[], "Cmd 1"=w411:string[], "Cmd 2"=w410:string[], "error out"=w418:errorcluster)  [unwired: 2 in, 2 out]
              "Loops Run" <- w394
            }
            frame #1 {
              w479 = FALSE ("Log (T)")
              n82 = call "WSVCAP SHL Host TL RFFE Configure.vi"("RFFE Slave Address"=w490, "Clock Rate (Hz)"=w488, "error in"=w480) -> ("Actual Rate (Hz)"=→"AR  Measurent(Hz)":dbl, "error out"=w486:errorcluster)  [unwired: 11 in]
              n83 = Array Size(array=w491) -> (size(s)=w500:i32)
              n84 = for {
                N: w500 -> [_]
                tunnel: w492 -> [w517]
                tunnel: [w501] -> w493
                tunnel: [w513] -> w474 mode=indexing
                tunnel: w491 -> [w515]
                tunnel: w486 -> [w503]
                tunnel: [w505] -> w485
                tunnel: w479 -> [w504]
                i -> [w512]
                stop <- w501 stop-if-true
                n85 = Index Array(array=w517, index=w512) -> (element=w516:string)
                n86 = Index Array(array=w515, index=w512) -> (element=w514:string)
                n87 = local write "STATUS"(w514) -> ()
                n88 = call "WSVCAP SHL Host TL RFFE Write - Multiple DUTs - Common Data.vi"("Data Out"=w516, "error in"=w503, "Log (T)"=FALSE) -> ("error out"=w507:errorcluster)  [unwired: 12 in]
                n89 = call "Delay.vi"("milliseconds to wait"=u32 10, "error in (no error)"=w507) -> ("error out"=w511:errorcluster)  [unwired: 9 in]
                n90 = call "WS1050 AD7747 READ 36 DUT.vi"("error in"=w511, "Log (T)"=w504, "DUT Mask Mode (All)"=WSVCAP_SHL_I2C_DUT_Mask_Mode_Enum."C1") -> ("error out"=w509:errorcluster, "AD7747 Values"=w510:string[][])  [unwired: 7 in]
                n91 = for {
                  tunnel: w510 -> [w520] mode=indexing
                  tunnel: w509 -> [w521]
                  tunnel: [w521] -> w505
                  tunnel: [w518] -> w513 mode=indexing
                  n92 = Index Array(array=w520, index=1) -> (element=w518:string)
                }
                n93 = Unbundle By Name(w505) -> ("status"=w501:bool)
              }
              n94 = Transpose 2D Array(2D array=w474) -> (transposed array=w484:string[][])
              "40V_1" <- w484
              "NOM IDD ON (uA)" <- w495
              "NOM IDD OFF(uA)" <- w494
            }
            frame #2 {
              n95 = Array Size(array=w540) -> (size(s)=w541:i32)
              n96 = for {
                N: w541 -> [_]
                tunnel: w539 -> [w567]
                tunnel: w538 -> [w565]
                tunnel: [w564] -> w537
                tunnel: [w560] -> w525 mode=indexing
                tunnel: w540 -> [w562]
                tunnel: w533 -> [w550]
                tunnel: [w552] -> w535
                tunnel: w527 -> [w551]
                i -> [w559]
                stop <- w564 stop-if-true
                n97 = Index Array(array=w567, index=w559) -> (element=w563:string)
                n98 = Index Array(array=w562, index=w559) -> (element=w561:string)
                n99 = call "WSVCAP SHL Host TL RFFE Write - Multiple DUTs - Common Data.vi"("Data Out"=w563, "error in"=w550, "Log (T)"=FALSE) -> ("error out"=w554:errorcluster)  [unwired: 12 in]
                n100 = local write "STATUS"(w561) -> ()
                n101 = call "Delay.vi"("milliseconds to wait"=u32 10, "error in (no error)"=w554) -> ("error out"=w558:errorcluster)  [unwired: 9 in]
                n102 = call "WS1050 AD7747 READ 36 DUT.vi"("error in"=w558, "Log (T)"=w551, "DUT Mask Mode (All)"=WSVCAP_SHL_I2C_DUT_Mask_Mode_Enum."C2") -> ("error out"=w556:errorcluster, "AD7747 Values"=w557:string[][])  [unwired: 7 in]
                n103 = for {
                  tunnel: w557 -> [w570] mode=indexing
                  tunnel: w556 -> [w571]
                  tunnel: [w571] -> w552
                  tunnel: [w568] -> w560 mode=indexing
                  n104 = Index Array(array=w570, index=3) -> (element=w568:string)
                }
                n105 = Unbundle By Name(w552) -> ("status"=w566:bool)
                n106 = Or(x=w566, y=w565) -> (x .or. y?=w564:bool)
              }
              n107 = Transpose 2D Array(2D array=w525) -> (transposed array=w534:string[][])
              "40V_2" <- w534
            }
            frame #3 {
              n108 = Array Size(array=w590) -> (size(s)=w591:i32)
              n109 = for {
                N: w591 -> [_]
                tunnel: w589 -> [w618]
                tunnel: w588 -> [w616]
                tunnel: [w615] -> w587
                tunnel: [w611] -> w576 mode=indexing
                tunnel: w590 -> [w613]
                tunnel: w582 -> [w601]
                tunnel: [w603] -> w575
                tunnel: w578 -> [w602]
                i -> [w610]
                stop <- w615 stop-if-true
                n110 = Index Array(array=w618, index=w610) -> (element=w614:string)
                n111 = Index Array(array=w613, index=w610) -> (element=w612:string)
                n112 = local write "STATUS"(w612) -> ()
                n113 = call "WSVCAP SHL Host TL RFFE Write - Multiple DUTs - Common Data.vi"("Data Out"=w614, "error in"=w601, "Log (T)"=FALSE) -> ("error out"=w605:errorcluster)  [unwired: 12 in]
                n114 = call "Delay.vi"("milliseconds to wait"=u32 10, "error in (no error)"=w605) -> ("error out"=w609:errorcluster)  [unwired: 9 in]
                n115 = call "WS1050 AD7747 READ 36 DUT.vi"("error in"=w609, "Log (T)"=w602, "DUT Mask Mode (All)"=WSVCAP_SHL_I2C_DUT_Mask_Mode_Enum."C3") -> ("error out"=w607:errorcluster, "AD7747 Values"=w608:string[][])  [unwired: 7 in]
                n116 = for {
                  tunnel: w608 -> [w621] mode=indexing
                  tunnel: w607 -> [w622]
                  tunnel: [w622] -> w603
                  tunnel: [w619] -> w611 mode=indexing
                  n117 = Index Array(array=w621, index=5) -> (element=w619:string)
                }
                n118 = Unbundle By Name(w603) -> ("status"=w617:bool)
                n119 = Or(x=w617, y=w616) -> (x .or. y?=w615:bool)
              }
              n120 = Transpose 2D Array(2D array=w576) -> (transposed array=w583:string[][])
              "40V_3" <- w583
            }
            frame #4 {
              # "VPI Testing @ 35V"
              n121 = call "WS1050 Delta C Calculation.vi"("error in (no error)"=w664, "DCap Target(pF)"=w663, "Input"=w666) -> ("error out"=w661:errorcluster, "Total Bank Delta C(pF)"=w654:string[], "% Bank DeltaC"=w658:string[])  [unwired: 4 in, 2 out]
              n122 = call "WS1050 Delta C Calculation.vi"("error in (no error)"=w664, "DCap Target(pF)"=w663, "Input"=w665) -> ("error out"=w662:errorcluster, "Total Bank Delta C(pF)"=w653:string[], "% Bank DeltaC"=w656:string[])  [unwired: 4 in, 2 out]
              n123 = call "WS1050 Delta C Calculation.vi"("error in (no error)"=w664, "DCap Target(pF)"=w663, "Input"=w657) -> ("error out"=w660:errorcluster, "Total Bank Delta C(pF)"=w652:string[], "% Bank DeltaC"=w655:string[])  [unwired: 4 in, 2 out]
              n124 = Merge Errors(w661, w662, w660) -> (w659:errorcluster)
              n125 = case shown="1, Default" w667 {
                tunnel: w659 -> [w696 w704]
                tunnel: [w696 w704] -> w626
                tunnel: w658 -> [w692 w700]
                tunnel: w656 -> [w691 w699]
                tunnel: w655 -> [w690 w698]
                tunnel: w654 -> [w695 w703]
                tunnel: [w695 w703] -> w651
                tunnel: w653 -> [w694 w702]
                tunnel: [w694 w702] -> w650
                tunnel: w652 -> [w693 w701]
                tunnel: [w693 w701] -> w649
                frame 0 {
                  n126 = Build Array(w692, w691, w690) -> (→"% Delta C_T0":string[][])
                }
                frame 1, Default {
                  n127 = Build Array(w700, w699, w698) -> (→"% Delta C":string[][])
                }
              }
              "Total Delta C1(pF)" <- w651
              "Total Delta C2(pF)" <- w650
              "Total Delta C3(pF)" <- w649
              n128 = call "WS1050_51 VPI Header.vi"("VPI Name"="VPI Name", "VPI_Cmd"="VPI_Cmd", "Cmin/Act"=w624, "WS1050/51"=w635, "error in (no error)"=w636) -> ("VPI_1"=w634:string[], "VPI_2"=w632:string[], "VPI Header"=w633:string[], "VPI_3"=w631:string[], "Cmd_3"=w628:string[], "Cmd_1"=w630:string[], "Cmd_2"=w629:string[], "error out"=w627:errorcluster)  [unwired: 3 in]
              n129 = Merge Errors(w627, w626) -> (w625:errorcluster)
              n130 = case shown="False" w641 {
                tunnel: w680 -> [w711 w749]
                tunnel: [w707 w727] -> w645
                tunnel: [w705 w751] -> w679
                tunnel: [w705 w735] -> w678
                tunnel: [w711 w733] -> w677
                tunnel: w674 -> [w713 w750]
                tunnel: [w713 w750] -> w673
                tunnel: w630 -> [_ w748]
                tunnel: w629 -> [_ w742]
                tunnel: w628 -> [_ w737]
                tunnel: [w705 w747] -> w670
                tunnel: w634 -> [w710 w745]
                tunnel: w632 -> [_ w743]
                tunnel: w631 -> [_ w738]
                tunnel: ["" ("string") w732] -> w647
                tunnel: w625 -> [w708 w724]
                frame False {
                  n131 = Array Size(array=w710) -> (size(s)=w709:i32)
                  n132 = for {
                    N: w709 -> [_]
                    tunnel: [w715] -> w706 mode=indexing
                    shift-right: [w714] -> w707
                    shift-left: w708 -> [w714]
                    n133 = for {
                      N: 36 -> [_]
                      tunnel: [""] -> w715 mode=indexing
                    }
                  }
                  n134 = Transpose 2D Array(2D array=w706) -> (transposed array=w705:string[][])
                  n135 = local write "VPI C1"(w705) -> ()
                  n136 = local write "VPI C2"(w705) -> ()
                  n137 = local write "VPI C3"(w705) -> ()
                }
                frame True {
                  w726 = FALSE ("Log (T)")
                  # "Set CP to 35V"
                  n138 = call "WSVCAP SHL Host TL RFFE Write - Multiple DUTs - Common Data.vi"("Data Out"="074820", "error in"=w724, "Log (T)"=w726) -> ("error out"=w722:errorcluster)  [unwired: 12 in]
                  n139 = call "Delay.vi"("milliseconds to wait"=u32 10, "error in (no error)"=w722) -> ("error out"=w728:errorcluster)  [unwired: 9 in]
                  n140 = case shown="3" "CP VPI" {
                    selector: "CP VPI" -> [w756 w761 w766 w770]
                    tunnel: string[] ["07476F", "074776", "074765", "074769", "07477B"] -> [w757 w762 w767 w772]
                    tunnel: [w755 w760 w765 w771] -> w720
                    tunnel: [w753 w758 w763 w768] -> w719
                    tunnel: ["35" ("string") "27.5" ("string") "30.5" ("string") "40.25" ("string")] -> w732
                    tunnel: w728 -> [w753 w758 w763 w768]
                    frame 0, Default {
                      n141 = Index Array(array=w757, index=w756) -> (element=w755:string)
                    }
                    frame 2 {
                      n142 = Index Array(array=w762, index=w761) -> (element=w760:string)
                    }
                    frame 3 {
                      n143 = Index Array(array=w767, index=w766) -> (element=w765:string)
                    }
                    frame 1 {
                      n144 = Index Array(array=w772, index=w770) -> (element=w771:string)
                    }
                  }
                  n145 = Array Size(array=w745) -> (size(s)=w752:i32)
                  n146 = call "WSVCAP SHL Host TL RFFE Write - Multiple DUTs - Common Data.vi"("Data Out"=w720, "error in"=w719, "Log (T)"=w726) -> ("error out"=w731:errorcluster)  [unwired: 12 in]
                  n147 = for {
                    N: w752 -> [_]
                    tunnel: w748 -> [w837]
                    tunnel: w749 -> [w835]
                    tunnel: [w834] -> w741
                    tunnel: [w832] -> w746 mode=indexing
                    tunnel: w745 -> [w831]
                    tunnel: w731 -> [w820]
                    tunnel: [w822] -> w730
                    i -> [w830]
                    stop <- w834 stop-if-true
                    n148 = Index Array(array=w837, index=w830) -> (element=w833:string)
                    n149 = Index Array(array=w831, index=w830) -> (element=w829:string)
                    n150 = local write "STATUS"(w829) -> ()
                    n151 = call "WSVCAP SHL Host TL RFFE Write - Multiple DUTs - Common Data.vi"("Data Out"=w833, "error in"=w820, "Log (T)"=FALSE) -> ("error out"=w828:errorcluster)  [unwired: 12 in]
                    n152 = call "Delay.vi"("milliseconds to wait"=u32 10, "error in (no error)"=w828) -> ("error out"=w824:errorcluster)  [unwired: 9 in]
                    n153 = call "WS1050 AD7747 READ 36 DUT.vi"("error in"=w824, "Log (T)"=FALSE, "DUT Mask Mode (All)"=WSVCAP_SHL_I2C_DUT_Mask_Mode_Enum."C1") -> ("error out"=w826:errorcluster, "AD7747 Values"=w825:string[][])  [unwired: 7 in]
                    n154 = for {
                      tunnel: [w840] -> w832 mode=indexing
                      tunnel: w826 -> [w839]
                      tunnel: [w839] -> w822
                      tunnel: w825 -> [w838] mode=indexing
                      n155 = Index Array(array=w838, index=1) -> (element=w840:string)
                    }
                    n156 = Unbundle By Name(w822) -> ("status"=w836:bool)
                    n157 = Or(x=w836, y=w835) -> (x .or. y?=w834:bool)
                  }
                  n158 = Transpose 2D Array(2D array=w746) -> (transposed array=w751:string[][])
                  "VPI C1" <- w751
                  n159 = Array Size(array=w743) -> (size(s)=w744:i32)
                  n160 = for {
                    N: w744 -> [_]
                    tunnel: w742 -> [w814]
                    tunnel: w741 -> [w812]
                    tunnel: [w811] -> w734
                    tunnel: [w809] -> w740 mode=indexing
                    tunnel: w743 -> [w808]
                    tunnel: w730 -> [w797]
                    tunnel: [w799] -> w729
                    i -> [w807]
                    stop <- w811 stop-if-true
                    n161 = Index Array(array=w814, index=w807) -> (element=w810:string)
                    n162 = Index Array(array=w808, index=w807) -> (element=w806:string)
                    n163 = call "WSVCAP SHL Host TL RFFE Write - Multiple DUTs - Common Data.vi"("Data Out"=w810, "error in"=w797, "Log (T)"=FALSE) -> ("error out"=w805:errorcluster)  [unwired: 12 in]
                    n164 = local write "STATUS"(w806) -> ()
                    n165 = call "Delay.vi"("milliseconds to wait"=u32 10, "error in (no error)"=w805) -> ("error out"=w801:errorcluster)  [unwired: 9 in]
                    n166 = call "WS1050 AD7747 READ 36 DUT.vi"("error in"=w801, "Log (T)"=FALSE, "DUT Mask Mode (All)"=WSVCAP_SHL_I2C_DUT_Mask_Mode_Enum."C2") -> ("error out"=w803:errorcluster, "AD7747 Values"=w802:string[][])  [unwired: 7 in]
                    n167 = for {
                      tunnel: [w817] -> w809 mode=indexing
                      tunnel: w803 -> [w816]
                      tunnel: [w816] -> w799
                      tunnel: w802 -> [w815] mode=indexing
                      n168 = Index Array(array=w815, index=3) -> (element=w817:string)
                    }
                    n169 = Unbundle By Name(w799) -> ("status"=w813:bool)
                    n170 = Or(x=w813, y=w812) -> (x .or. y?=w811:bool)
                  }
                  n171 = Transpose 2D Array(2D array=w740) -> (transposed array=w747:string[][])
                  "VPI C2" <- w747
                  n172 = Array Size(array=w738) -> (size(s)=w739:i32)
                  n173 = for {
                    N: w739 -> [_]
                    tunnel: w737 -> [w791]
                    tunnel: w734 -> [w789]
                    tunnel: [w788] -> w733
                    tunnel: [w786] -> w736 mode=indexing
                    tunnel: w738 -> [w785]
                    tunnel: w729 -> [w774]
                    tunnel: [w776] -> w727
                    i -> [w784]
                    stop <- w788 stop-if-true
                    n174 = Index Array(array=w791, index=w784) -> (element=w787:string)
                    n175 = Index Array(array=w785, index=w784) -> (element=w783:string)
                    n176 = call "WSVCAP SHL Host TL RFFE Write - Multiple DUTs - Common Data.vi"("Data Out"=w787, "error in"=w774, "Log (T)"=FALSE) -> ("error out"=w782:errorcluster)  [unwired: 12 in]
                    n177 = local write "STATUS"(w783) -> ()
                    n178 = call "Delay.vi"("milliseconds to wait"=u32 10, "error in (no error)"=w782) -> ("error out"=w778:errorcluster)  [unwired: 9 in]
                    n179 = call "WS1050 AD7747 READ 36 DUT.vi"("error in"=w778, "Log (T)"=FALSE, "DUT Mask Mode (All)"=WSVCAP_SHL_I2C_DUT_Mask_Mode_Enum."C3") -> ("error out"=w780:errorcluster, "AD7747 Values"=w779:string[][])  [unwired: 7 in]
                    n180 = for {
                      tunnel: [w794] -> w786 mode=indexing
                      tunnel: w780 -> [w793]
                      tunnel: [w793] -> w776
                      tunnel: w779 -> [w792] mode=indexing
                      n181 = Index Array(array=w792, index=5) -> (element=w794:string)
                    }
                    n182 = Unbundle By Name(w776) -> ("status"=w790:bool)
                    n183 = Or(x=w790, y=w789) -> (x .or. y?=w788:bool)
                  }
                  n184 = Transpose 2D Array(2D array=w736) -> (transposed array=w735:string[][])
                  "VPI C3" <- w735
                }
              }
              n185 = Insert Into Array(array=w669, new element=w633) -> (w668:string[])  [unwired: 1 in]
              n186 = case shown="True" w646 {
                tunnel: w645 -> [w682 w687]
                tunnel: [w683 w686] -> w644
                frame False {
                  n187 = call "WSVCAP SHL Host TL RFFE Write - Multiple DUTs - Common Data.vi"("Data Out"="074820", "error in"=w682, "Log (T)"=FALSE) -> ("error out"=w683:errorcluster)  [unwired: 12 in]
                }
                frame True {
                  n188 = call "WSVCAP SHL Host TL RFFE Write - Multiple DUTs - Common Data.vi"("Data Out"="074800", "error in"=w687, "Log (T)"=FALSE) -> ("error out"=w686:errorcluster)  [unwired: 12 in]
                }
              }
              n189 = call "Delay.vi"("milliseconds to wait"=u32 10, "error in (no error)"=w644) -> ("error out"=w643:errorcluster)  [unwired: 9 in]
            }
            frame #5 {
              # "VSA Testing"
              n190 = case shown="False" w843 {
                tunnel: w881 -> [w893 w907]
                tunnel: [w892 w906] -> w856
                tunnel: [w897 w913] -> w872
                tunnel: w873 -> [w897 w912]
                tunnel: [w894 w910] -> w861
                tunnel: [w894 w909] -> w858
                tunnel: [w894 w908] -> w855
                tunnel: [w895 w911] -> w862
                frame False {
                  n191 = for {
                    tunnel: dbl[] [0.0, 0.0, 0.0] -> [w902] mode=indexing
                    tunnel: [w901] -> w895 mode=indexing
                    tunnel: [w898] -> w894 mode=indexing
                    shift-right: [w899] -> w892
                    shift-left: w893 -> [w899]
                    n192 = Number To Fractional String(number=w902) -> (F-format string=w903:string)  [unwired: 3 in]
                    n193 = for {
                      N: 36 -> [_]
                      tunnel: w903 -> [w905]
                      tunnel: [w905] -> w901 mode=indexing
                      tunnel: [""] -> w898 mode=indexing
                    }
                  }
                }
                frame True {
                  n194 = for {
                    tunnel: "VSA Voltage(V)" -> [w937] mode=indexing
                    tunnel: [w941] -> w913
                    tunnel: w912 -> [w939]
                    tunnel: [w938] -> w910 mode=indexing
                    tunnel: [w925] -> w909 mode=indexing
                    tunnel: [w934] -> w911 mode=indexing
                    tunnel: [w919] -> w908 mode=indexing
                    tunnel: w907 -> [w918]
                    tunnel: [w917] -> w906
                    w916 = FALSE ("Log (T)")
                    w933 = u16 0 items=["Voltage", "Current"] ("Source Mode  (0: Voltage)")
                    n195 = call "Ke2400 Configure Output.vi"("Source Mode  (0: Voltage)"=w933, "error in (no error)"=w918, "Compliance  Level (0.1)"=0.1, "Output Level (0)"=w937, "VISA resource name"=w939) -> ("error out"=w945:errorcluster, "VISA resource name out"=w943:refnum<visa-resource-name>)  [unwired: 5 in]
                    n196 = call "Ke2400 Enable.vi"("error in (no error)"=w945, "ON/OFF"=TRUE ("Enable Output (T: Enable)"), "VISA resource name"=w943) -> ("error out"=w946:errorcluster, "VISA resource name out"=w941:refnum<visa-resource-name>)  [unwired: 7 in]
                    n197 = call "Delay.vi"("milliseconds to wait"=u32 10, "error in (no error)"=w946) -> ("error out"=w932:errorcluster)  [unwired: 9 in]
                    n198 = call "WS1050 AD7747 READ 36 DUT.vi"("error in"=w932, "Log (T)"=w916, "DUT Mask Mode (All)"=WSVCAP_SHL_I2C_DUT_Mask_Mode_Enum."C1") -> ("error out"=w929:errorcluster, "AD7747 Values"=w931:string[][])  [unwired: 7 in]
                    n199 = for {
                      tunnel: w931 -> [w957] mode=indexing
                      tunnel: [w958] -> w938 mode=indexing
                      tunnel: w929 -> [w956]
                      tunnel: [w956] -> w928
                      n200 = Index Array(array=w957, index=1) -> (element=w958:string)
                    }
                    n201 = call "WS1050 AD7747 READ 36 DUT.vi"("error in"=w928, "Log (T)"=w916, "DUT Mask Mode (All)"=WSVCAP_SHL_I2C_DUT_Mask_Mode_Enum."C2") -> ("error out"=w926:errorcluster, "AD7747 Values"=w924:string[][])  [unwired: 7 in]
                    n202 = for {
                      tunnel: w924 -> [w952] mode=indexing
                      tunnel: [w953] -> w925 mode=indexing
                      tunnel: w926 -> [w951]
                      tunnel: [w951] -> w923
                      n203 = Index Array(array=w952, index=3) -> (element=w953:string)
                    }
                    n204 = Number To Fractional String(number=w937) -> (F-format string=w936:string)  [unwired: 3 in]
                    n205 = call "WS1050 AD7747 READ 36 DUT.vi"("error in"=w923, "Log (T)"=w916, "DUT Mask Mode (All)"=WSVCAP_SHL_I2C_DUT_Mask_Mode_Enum."C3") -> ("error out"=w921:errorcluster, "AD7747 Values"=w920:string[][])  [unwired: 7 in]
                    n206 = for {
                      tunnel: w920 -> [w948] mode=indexing
                      tunnel: [w949] -> w919 mode=indexing
                      tunnel: w921 -> [w947]
                      tunnel: [w947] -> w917
                      n207 = Index Array(array=w948, index=5) -> (element=w949:string)
                    }
                    n208 = for {
                      N: 36 -> [_]
                      tunnel: w936 -> [w955]
                      tunnel: [w955] -> w934 mode=indexing
                    }
                  }
                  n209 = local write "STATUS"("VSA Testing...." ("STATUS")) -> ()
                }
              }
              n210 = Transpose 2D Array(2D array=w862) -> (transposed array=w860:string[][])
              n211 = Transpose 2D Array(2D array=w861) -> (transposed array=w859:string[][])
              n212 = Transpose 2D Array(2D array=w858) -> (transposed array=w857:string[][])
              n213 = Transpose 2D Array(2D array=w855) -> (transposed array=w854:string[][])
              n214 = call "WS1050_VSA_Convert_Data.vi"("VSA_C3"=w854, "error in (no error)"=w856, "VSA_C2"=w857, "VSA_C1"=w859, "Voltage"=w860) -> ("error out"=w853:errorcluster, "VSA_V3"=w850:string[][], "VSA_V2"=w851:string[][], "VSA_V1"=w852:string[][])  [unwired: 3 in]
              "VSA_V1" <- w852
              "VSA_V2" <- w851
              "VSA_V3" <- w850
              n215 = case shown="True" w843 {
                tunnel: w872 -> [w885 w891]
                tunnel: [w885 w890] -> w871
                tunnel: w853 -> [w884 w889]
                tunnel: [w884 w886] -> w870
                frame False {
                }
                frame True {
                  w887 = u16 0 items=["Voltage", "Current"] ("Source Mode  (0: Voltage)")
                  n216 = call "Ke2400 Configure Output.vi"("Source Mode  (0: Voltage)"=w887, "error in (no error)"=w889, "Output Level (0)"=0.0, "VISA resource name"=w891) -> ("error out"=w886:errorcluster, "VISA resource name out"=w890:refnum<visa-resource-name>)  [unwired: 6 in]
                }
              }
              n217 = call "Delay.vi"("milliseconds to wait"=u32 50, "error in (no error)"=w870) -> ("error out"=w869:errorcluster)  [unwired: 9 in]
            }
            frame #6 {
              # "Handshake Check and EFuse Readback"
              n218 = Or(x=w971, y=w977) -> (x .or. y?=w976:bool)
              n219 = case shown="False" w976 {
                tunnel: w999 -> [w1012 _]
                tunnel: w998 -> [w1011 w1016]
                tunnel: [w1010 w1015] -> w997
                tunnel: w996 -> [w1009 _]
                tunnel: w995 -> [w1008 _]
                tunnel: w994 -> [w1007 _]
                tunnel: [w1003 w1018] -> w993
                tunnel: [w1002 w1018] -> w988
                tunnel: w961 -> [w1001 _]
                tunnel: w982 -> [w1000 _]
                frame False {
                  n220 = call "WS1050_36DUT_Handshake Check R1_Record All Regs Ver1.0.vi"("file path (use dialog)"=w1012, "Reg1_Bit Cntrl"="Reg1_Bit Cntrl", "File Name"=w1000, "SN"=w1007, "Loop"=w1001, "error"=w1011, "Lot #"=w1009, "Wafer #"=w1008) -> ("Pass/Fail"=→"EFuse Readback Status":bool[], "EFuse Read back"=w1002:string[], "Status"=w1003:string[], "error out"=w1010:errorcluster)  [unwired: 6 in, 2 out]
                  n221 = case shown="1, Default" w1001 {
                    tunnel: w1002 -> [w1013 w1014]
                    frame 0 {
                      "EFuse RB T0" <- w1013
                    }
                    frame 1, Default {
                      "Current EFuse Read back" <- w1014
                    }
                  }
                  n222 = local write "STATUS"("Hand Shake & EFuse Readback...." ("STATUS")) -> ()
                }
                frame True {
                  n223 = for {
                    N: 36 -> [_]
                    tunnel: [""] -> w1018 mode=indexing
                    tunnel: w1016 -> [w1019]
                    tunnel: [w1019] -> w1015
                  }
                }
              }
              n224 = Build Array(w986, w984, w983) -> (w985:string[])
            }
            frame #7 {
              # "Save Data"
              n225 = Increment(x=w1033) -> (x+1=w1021:i32)
              n226 = local write "STATUS"("Saving Data...." ("STATUS")) -> ()
              n227 = Multiply(x=w1021, y=36) -> (x*y=w1029:i32)
              n228 = Path To String(path=w1037) -> (string=w1036:string)
              n229 = Bundle("Test Program"=w1066, "Comment"=w1065, "Data Out"=w1044, "Data Out"=w1043, "CP Voltage"=w1042, w1041, "% Duty Cycle"=w1040, "CP Voltage"=w1039, "string"=w1038, "Freq(Hz)"=w1027, "Board#"=w1025) -> (w1026:T6)  [unwired: 1 in]
              n230 = case shown="False" w1022 {
                tunnel: w1029 -> [w1073 w1076]
                tunnel: [w1073 w1074] -> w1028
                frame False {
                }
                frame True {
                  n231 = Multiply(x=w1076, y="No of Rows\nFrom Spread Sheet") -> (x*y=w1074:i32)
                }
              }
              n232 = call "WS1050_36 DUT SData Ver1.0.vi"("TMN DC\\CAP Data Log File Path"=w1037, "Lot#"=w1068, "Total Delta C1(pF)"=w1047, "VSA_V1"=w1055, "Wafer#"=w1064, "File Name"=w1031, "Total Delta C2(pF)"=w1046, "error in"=w1071, "TP/Comment"=w1026, "EFuse"=w1058, "Data Output C3"=w1049, "Temperature"=w1053, "VSA_V2"=w1056, "VPI C3"=w1051, "Data Output C1"=w1061, "VPI C2"=w1050, "SN"=w1069, "R/W Status"=w1067, "Cap Header"=w1052, "HD/Cycles Completed"="HD/Cycles Completed", "Data Output C2"=w1048, "VSA_V3"=w1054, "Current"=w1060, "VPI C1"=w1059, "Total Delta C3(pF)"=w1045) -> ("error out"=w1070:errorcluster)  [unwired: 2 in]
              n233 = Concatenate Strings(w1036, "\\" ("string"), w1031, "_Multi Socket Data.csv" ("string")) -> (w1035:string)
            }
            frame #8 {
              n234 = case shown="True" "Plot Delta Cmin" {
                tunnel: w1085 -> [w1094 w1109]
                tunnel: [w1094 w1105] -> w1084
                tunnel: w1083 -> [_ w1101]
                tunnel: w1081 -> [_ w1099]
                frame False {
                }
                frame True {
                  n235 = String To Path(string=w1101) -> (path=w1100:path)
                  n236 = call "Delay.vi"("milliseconds to wait"=u32 50, "error in (no error)"=w1109) -> ("error out"=w1108:errorcluster)  [unwired: 9 in]
                  n237 = call "36DUT Plot From Spread Sheet.vi"("Plot"="Plot", "No of Rows"=w1099, "error in (no error)"=w1108, "Bank"="Bank", "file path (dialog if empty)"=w1100) -> ("error out"=w1103:errorcluster, "Delta C_Min Plot"=→"Plot_1":dbl[][])  [unwired: 5 in]
                  n238 = call "36DUT Plot From Spread Sheet.vi"("Plot"="Plot", "No of Rows"=w1099, "error in (no error)"=w1103, "Bank"="Bank 2", "file path (dialog if empty)"=w1100) -> ("error out"=w1104:errorcluster, "Delta C_Min Plot"=→"Plot_2":dbl[][])  [unwired: 5 in]
                  n239 = call "36DUT Plot From Spread Sheet.vi"("Plot"="Plot", "No of Rows"=w1099, "error in (no error)"=w1104, "Bank"="Bank 3", "file path (dialog if empty)"=w1100) -> ("error out"=w1105:errorcluster, "Delta C_Min Plot"=→"Plot_3":dbl[][])  [unwired: 5 in]
                }
              }
              n240 = Increment(x=w1078) -> (x+1=w1077:i32)
              "No of HD/Cycle\nCompleted" <- w1077
              n241 = Get Date/Time In Seconds() -> (seconds since 1Jan1904=w1087:timestamp)
              n242 = Get Date/Time String(seconds (now)=w1087, want seconds? (F)=TRUE) -> (date string=→"date string":string, time string=→"Previous Time":string)  [unwired: 1 in]
              n243 = local write "RB Reg for HD/Cycle"(string[] []) -> ()
              n244 = Greater Or Equal?(x=w1077, y=w1080) -> (x >= y?=w1091:bool)
            }
          }
          n245 = call "Delay.vi"("milliseconds to wait"=u32 10, "error in (no error)"=w225) -> ("error out"=w226:errorcluster)  [unwired: 9 in]
          n246 = Compound Arithmetic op=OR(w377, w297) -> (w326:bool)
          "Loop \ncompleted" <- w169
        }
        n247 = local write "No of HD/Cycle\nCompleted"(u64 0 ("No of HD/Cycle\nCompleted")) -> ()
        n248 = Unbundle By Name(w151) -> ("status"=w157:bool)
        n249 = Compound Arithmetic op=OR(w157, w155) -> (w141:bool)
      }
      n250 = VISA Write(VISA resource name=w65, write buffer="SOUR:FUNC VOLT;VOLT:MODE FIX;RANG 100;LEV 0.0;:SENS:FUNC \"CURR\";CURR:PROT 60E-3;RANG 100E-3;:OUTP ON", error in (no error)=w50) -> (VISA resource name out=w64:refnum<visa-resource-name>, error out=w28:errorcluster)  [unwired: 1 out]
    }
  }
  "Ke2000 Out" <- w22
  "PS1 Out" <- w21
  "Ke2400 Out" <- w16
  "error out" <- w15
  "STATUS" <- "Idle...." ("STATUS")
